vi "IsNumeric.vi"(4 "Value String in":string) -> (0 "IsNumeric":bool, 2 "Numeric Value":dbl)   [LabVIEW 2019]
uses:
  <vilib>/regexp/Match Regular Expression.xnode
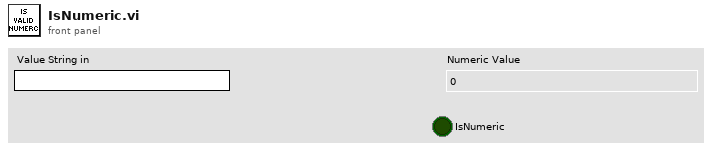
[diagram p1: front panel]
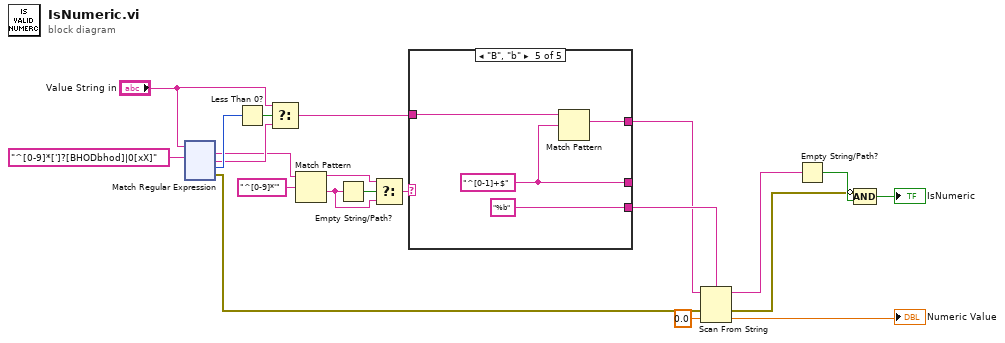
[diagram p0: block diagram]
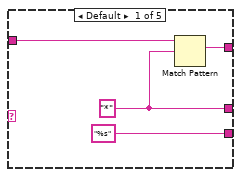
[diagram p2: hidden frame]
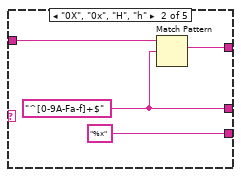
[diagram p3: hidden frame]
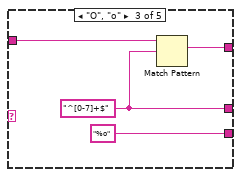
[diagram p4: hidden frame]
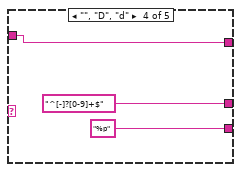
[diagram p5: hidden frame]
diagram:
  n1 = xnode ("Match Regular Expression")("input string"="Value String in", "regular expression"="^[0-9]*[']?[BHODbhod]|0[xX]") -> ("whole match"=w16:string, "after match"=w19:string, "offset past match"=w21:i32, "error out"=w9:errorcluster)  [unwired: 4 in, 1 out]
  n2 = Less Than 0?(x=w21) -> (x < 0?=w20:bool)
  n3 = Select(t="Value String in", s=w20, f=w19) -> (s? t:f=w6:string)
  n4 = Match Pattern(string=w16, regular expression="^[0-9]*'") -> (before substring=w13:string, after substring=w14:string)  [unwired: 1 in, 2 out]
  n5 = Empty String/Path?(string/path=w14) -> (empty?=w15:bool)
  n6 = Select(t=w13, s=w15, f=w14) -> (s? t:f=w12:string)
  n7 = case shown="\"B\", \"b\"" w12 {
    tunnel: ["%s" ("format string") "%x" ("format string") "%o" ("format string") "%p" ("format string") "%b" ("format string")] -> w11
    tunnel: [w23 w27 w31 "^[-]?[0-9]+$" ("format string") w38] -> _
    tunnel: w6 -> [w24 w28 w32 w34 w39]
    tunnel: [w22 w26 w30 w34 w37] -> w5
    frame Default {
      w23 = "*" ("format string")
      n8 = Match Pattern(string=w24, regular expression=w23) -> (match substring=w22:string)  [unwired: 1 in, 3 out]
    }
    frame "0X", "0x", "H", "h" {
      w27 = "^[0-9A-Fa-f]+$" ("format string")
      n9 = Match Pattern(string=w28, regular expression=w27) -> (match substring=w26:string)  [unwired: 1 in, 3 out]
    }
    frame "O", "o" {
      w31 = "^[0-7]+$" ("format string")
      n10 = Match Pattern(string=w32, regular expression=w31) -> (match substring=w30:string)  [unwired: 1 in, 3 out]
    }
    frame "", "D", "d" {
    }
    frame "B", "b" {
      w38 = "^[0-1]+$" ("format string")
      n11 = Match Pattern(string=w39, regular expression=w38) -> (match substring=w37:string)  [unwired: 1 in, 3 out]
    }
  }
  n12 = Scan From String(format string=w11, input string=w5, error in=w9, default 1=0.0 ("number")) -> (remaining string=w2:string, error out=w3:errorcluster, output 1=→"Numeric Value":dbl)  [unwired: 1 in, 1 out]
  n13 = Empty String/Path?(string/path=w2) -> (empty?=w4:bool)
  n14 = Compound Arithmetic op=AND(invert w3, w4) -> (→"IsNumeric":bool)
